vi "SbigDll.vi"(0 "error in (no error)":errorcluster, 2 "Command":T1(ring), 5 "Results In":u16[](array[numeric])=[0], 6 "Parameters":u16[](array[numeric])=[0]) -> (3 "error out":errorcluster, 4 "Status":bool, 7 "Results Out":u16[](array[numeric]))   [LabVIEW 2009]
uses:
  Program Files/SBIG/Driver Checker/SBIG Drivers/SBIGUDrv.dll
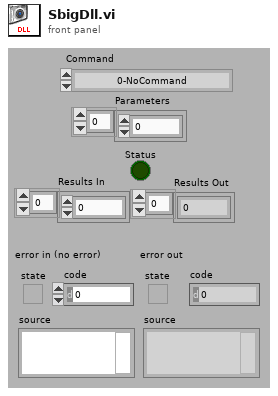
[diagram p1: front panel]
types:
  T1 = enum16{"0-NoCommand", "1-StartExposure", "2-EndExposure", "3-ReadoutLine", "4-DumpLines", "5-SetTemperatureRegulation", "6-QueryTemperatureStatus", "7-ActivateRelay", "8-PulseOut", "9-EstablishLink", "10-GetDriverInfo", "11-GetCCDInfo", "12-QueryCommandStatus", "13-MiscellaneousControl", "14-ReadSubstractLine", "15-UpdateClock", "16-ReadOffset", "17-OpenDriver", "18-CloseDriver", "19-TXSerialBytes", "20-GetSerialStatus", "21-AOTipTilt", "22-AOSetFocus", "23-AODelay", "24-GetTurboStatus", "25-EndReadout", "26-GetUSTimer", "27-OpenDevice", "28-CloseDevice", "29-SetIRQL", "30-GetIRQL", "31-GetLine", "32-GetLinkStatus", "33-GetDriverHandle", "34-SetDriverHandle", "35-StartReadout", "36-GetErrorString", "37-SetDriverControl", "38-GetDriverControl", "39-USBADControl", "40-QueryUSB", "41-GetPentiumCycleCount", "42-RWUSBI2C", "43-CFW"}
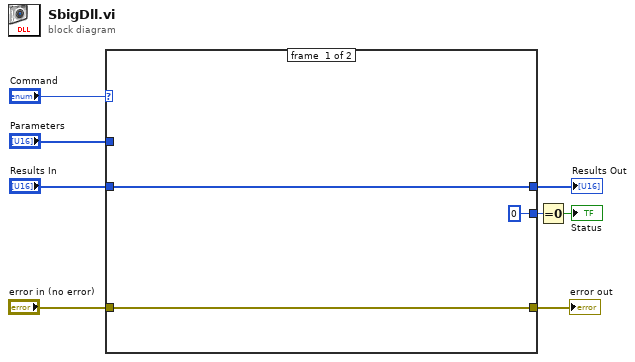
[diagram p0: block diagram]
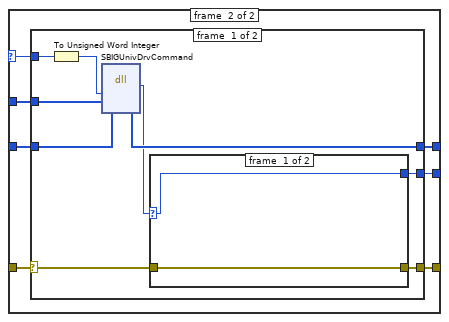
[diagram p2: hidden frame]
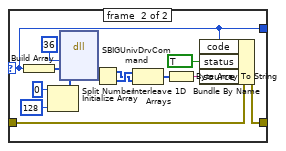
[diagram p3: hidden frame]
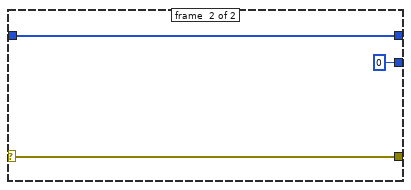
[diagram p4: hidden frame]
diagram:
  n1 = case shown="\"1-StartExposure\", Default" "Command" {
    selector: "Command" -> [_ w15]
    tunnel: "Parameters" -> [_ w18]
    tunnel: "Results In" -> [w11 w17]
    tunnel: [w11 w16] -> w6
    tunnel: "error in (no error)" -> [w10 w13]
    tunnel: [w10 w14] -> w4
    tunnel: [u16 0 w12] -> w2
    frame #0 {
    }
    frame #1 {
      n2 = case shown="No Error" w13 {
        selector: w13 -> [w22 w46]
        tunnel: w18 -> [w27 _]
        tunnel: w17 -> [w26 w45]
        tunnel: [w25 w45] -> w16
        tunnel: w15 -> [w24 _]
        tunnel: [w23 w46] -> w14
        tunnel: [w19 u16 0] -> w12
        frame #0 {
          n3 = To Unsigned Word Integer(number=w24) -> (unsigned 16bit integer=w20:u16)
          n4 = dll-call lib="D:/Program Files/SBIG/Driver Checker/SBIG Drivers/SBIGUDrv.dll" fn="SBIGUnivDrvCommand"("Command"=w20, "Parameters"=w27, "Results"=w26) -> (w21:u16, "Results"=w25:u16[])  [unwired: 5 in, 2 out]
          n5 = case shown="1, Default" w21 {
            selector: w21 -> [w28 w30]
            tunnel: w22 -> [w29 w38]
            tunnel: [w29 w37] -> w23
            tunnel: [w28 w30] -> w19
            frame #0 {
            }
            frame #1 {
              n6 = Build Array(w30) -> (w42:u16[])
              n7 = Initialize Array(u16 0 ("Nouvel élément"), 128 ("Taille de la dimension")) -> (w41:u16[])
              n8 = dll-call lib="D:/Program Files/SBIG/Driver Checker/SBIG Drivers/SBIGUDrv.dll" fn="SBIGUnivDrvCommand"("Command"=u16 36, "Parameters"=w42, "Results"=w41) -> ("Results"=w34:u16[])  [unwired: 5 in, 3 out]
              n9 = Split Number(x=w34) -> (hi(x)=w31:u8[], lo(x)=w32:u8[])
              n10 = Interleave 1D Arrays(w32, w31) -> (w33:u8[])
              n11 = Byte Array To String(unsigned byte array=w33) -> (string=w36:string)
              n12 = Bundle By Name(cluster=w38, "code"=w30, "status"=TRUE, "source"=w36) -> (w37:errorcluster)
            }
          }
        }
        frame #1 {
        }
      }
    }
  }
  "error out" <- w4
  "Results Out" <- w6
  n13 = Equal To 0?(x=w2) -> (x = 0?=→"Status":bool)
